vi "AddFavList.vi"(11 "Tags":T1={"Pattern (eg. H,V)"="", "File type"={"AvR"=TRUE, "AvC"=FALSE, "trf"=FALSE, "wfm"=FALSE, "All"=FALSE}, "Tags 1"="", "Tags 2"="", "Tags 3"=""}) -> (0 "Extensions":string[](array[string]), 1 "Paths from lists":path[](array[path]), 3 "Tags":string[](array[string]))   [LabVIEW 2022 SP3]
uses:
  <vilib>/Utility/error.llb/Trim Whitespace One-Sided.vi
panel:
  # "Or"
  # "Or"
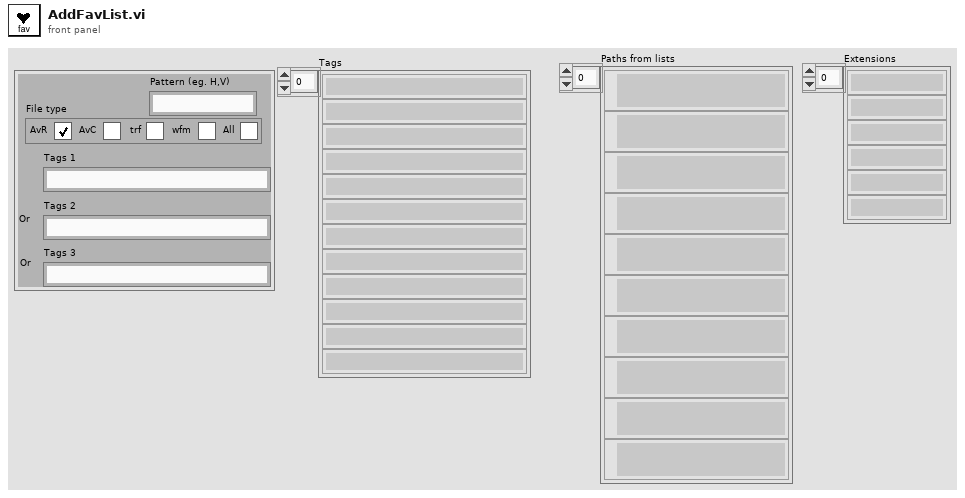
[diagram p1: front panel]
types:
  T1 = cluster{"Pattern (eg. H,V)":string, "File type":cluster{"AvR":bool, "AvC":bool, "trf":bool, "wfm":bool, "All":bool}, "Tags 1":string, "Tags 2":string, "Tags 3":string}
  T2 = cluster{"AvR":bool, "AvC":bool, "trf":bool, "wfm":bool, "All":bool}
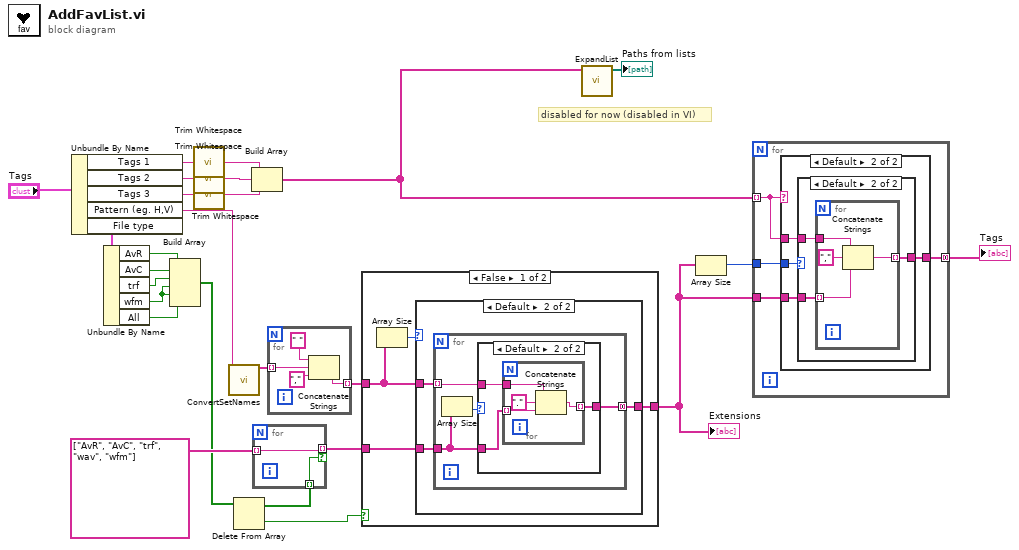
[diagram p0: block diagram]
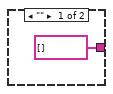
[diagram p2: hidden frame]
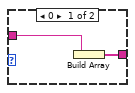
[diagram p3: hidden frame]
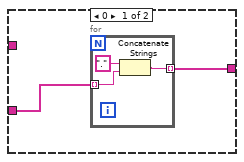
[diagram p4: hidden frame]
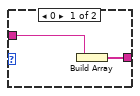
[diagram p5: hidden frame]
diagram:
  # "disabled for now (disabled in VI)"
  n1 = Unbundle By Name("Tags") -> ("Tags 1"=w23:string, "Tags 2"=w24:string, "Tags 3"=w25:string, "Pattern (eg. H,V)"=w13:string, "File type"=w11:T2)
  n2 = Unbundle By Name(w11) -> ("AvR"=w10:bool, "AvC"=w9:bool, "trf"=w8:bool, "wfm"=w7:bool, "All"=w6:bool)
  n3 = Build Array(w10, w9, w8, w7, w7, w6) -> (w5:bool[])
  n4 = call <vilib>:"Trim Whitespace.vi"("string"=w23) -> ("trimmed string"=w4:string)  [unwired: 1 in]
  n5 = call <vilib>:"Trim Whitespace.vi"("string"=w24) -> ("trimmed string"=w3:string)  [unwired: 1 in]
  n6 = call <vilib>:"Trim Whitespace.vi"("string"=w25) -> ("trimmed string"=w2:string)  [unwired: 1 in]
  n7 = call "ConvertSetNames.vi"("Set Names"=w13) -> ("Set Names"=w1:string[])  [unwired: 10 in]
  n8 = Delete From Array(array=w5) -> (deleted portion=w19:bool, array with subset deleted=w22:bool[])  [unwired: 2 in]
  n9 = Build Array(w4, w3, w2) -> (w14:string[])
  n10 = for {
    tunnel: [w28] -> w20 mode=indexing if=w27
    tunnel: string[] ["AvR", "AvC", "trf", "wav", "wfm"] -> [w28] mode=indexing
    tunnel: w22 -> [w27] mode=indexing
  }
  n11 = for {
    tunnel: [w32] -> w12 mode=indexing
    tunnel: w1 -> [w30] mode=indexing
    n12 = Concatenate Strings(" ", w30, ",") -> (w32:string)
  }
  n13 = case shown="False" w19 {
    tunnel: [w36 w58] -> w16
    tunnel: w12 -> [w34 w58]
    tunnel: w20 -> [w35 _]
    frame False {
      n14 = Array Size(array=w34) -> (size(s)=w33:i32)
      n15 = case shown="Default" w33 {
        tunnel: [w37 w44] -> w36
        tunnel: w35 -> [w38 w43]
        tunnel: w34 -> [_ w42]
        frame 0 {
          n16 = for {
            tunnel: w38 -> [w40] mode=indexing
            tunnel: [w39] -> w37 mode=indexing
            n17 = Concatenate Strings("." ("string"), w40) -> (w39:string)
          }
        }
        frame Default {
          n18 = for {
            tunnel: w42 -> [w48] mode=indexing
            tunnel: w43 -> [w46]
            tunnel: [w47] -> w44 mode=concatenating
            n19 = Array Size(array=w46) -> (size(s)=w45:i32)
            n20 = case shown="Default" w45 {
              tunnel: w46 -> [_ w53]
              tunnel: w48 -> [w50 w52]
              tunnel: [w49 w51] -> w47
              frame 0 {
                n21 = Build Array(w50) -> (w49:string[])
              }
              frame Default {
                n22 = for {
                  tunnel: w53 -> [w57] mode=indexing
                  tunnel: w52 -> [w55]
                  tunnel: [w56] -> w51 mode=indexing
                  n23 = Concatenate Strings(w55, "." ("string"), w57) -> (w56:string)
                }
              }
            }
          }
        }
      }
    }
    frame True {
    }
  }
  "Extensions" <- w16
  n24 = call "ExpandList.vi"("Tags in"=w14) -> ("List Paths"=→"Paths from lists":path[])  [unwired: 9 in, 1 out]
  n25 = Array Size(array=w16) -> (size(s)=w17:i32)
  n26 = for {
    tunnel: w14 -> [w61] mode=indexing
    tunnel: w17 -> [w62]
    tunnel: w16 -> [w60]
    tunnel: [w59] -> w15 mode=concatenating
    n27 = case shown="Default" w61 {
      tunnel: w62 -> [_ w67]
      tunnel: w61 -> [_ w66]
      tunnel: w60 -> [_ w65]
      tunnel: [string[] [] w64] -> w59
      frame "" {
      }
      frame Default {
        n28 = case shown="Default" w67 {
          tunnel: w66 -> [w69 w72]
          tunnel: w65 -> [_ w71]
          tunnel: [w68 w70] -> w64
          frame 0 {
            n29 = Build Array(w69) -> (w68:string[])
          }
          frame Default {
            n30 = for {
              tunnel: w72 -> [w76]
              tunnel: w71 -> [w74] mode=indexing
              tunnel: [w73] -> w70 mode=indexing
              n31 = Concatenate Strings(w76, "," ("string"), w74) -> (w73:string)
            }
          }
        }
      }
    }
  }
  "Tags" <- w15
